vi "Construct.vi"(8 "error in (no error)":errorcluster, 9 "Launch Type (0)":i32, 10 "Default Path":path, 11 "StatusQueue":refnum<queue>) -> (0 "error out":errorcluster, 3 "Controller out":refnum<class "Controller.lvclass">)   [LabVIEW 2013, in "SET Project Editor.lvlib" / "Controller.lvclass"]
uses:
  Controller.lvclass
  Controller.lvclass/Controller.ctl
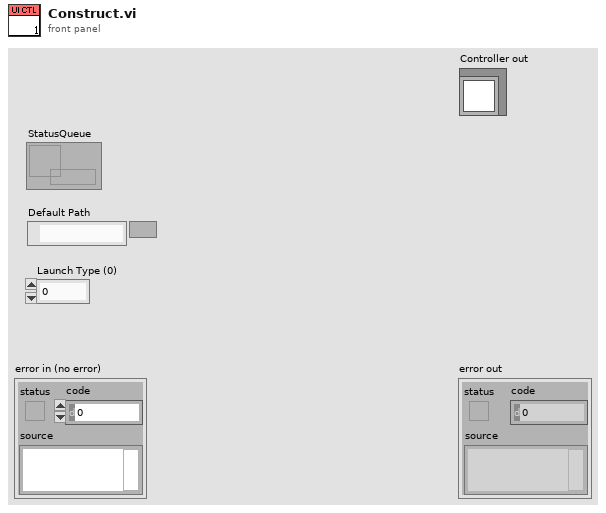
[diagram p1: front panel]
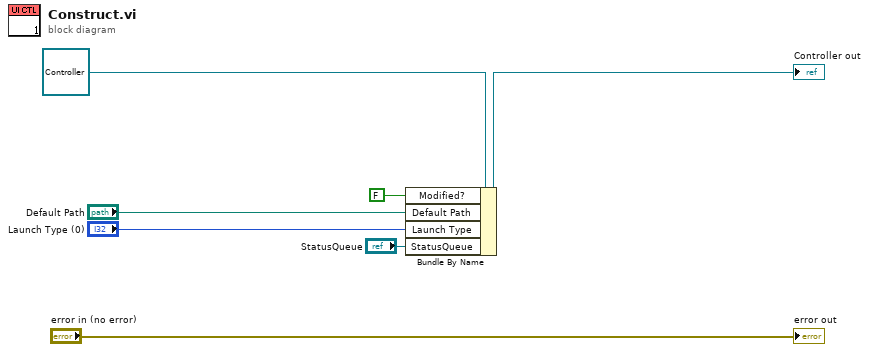
[diagram p0: block diagram]
diagram:
  n1 = Bundle By Name(cluster=refnum<class "Controller.lvclass"> refnum ("Controller in"), "Modified?"=FALSE, "Default Path"="Default Path", "Launch Type"="Launch Type (0)", "StatusQueue"="StatusQueue") -> (→"Controller out":refnum<class "Controller.lvclass">)
  "error out" <- "error in (no error)"
